vi "CreateFolder.vi"(4 "error in (no error)":errorcluster caption="エラー入力(エラーなし)", 7 "パス":path) -> (0 "error out":errorcluster caption="エラー出力", 3 "パス出力":path)   [LabVIEW 2015]
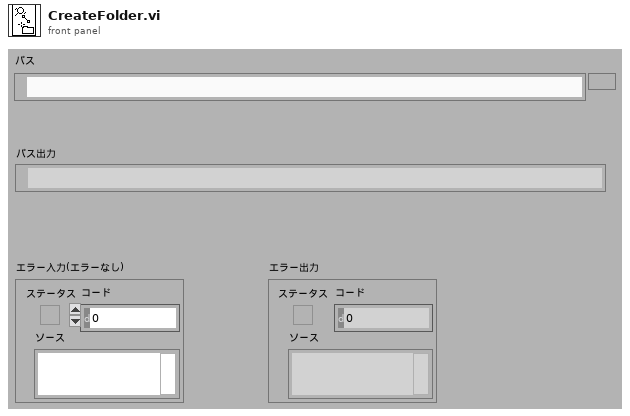
[diagram p1: front panel]
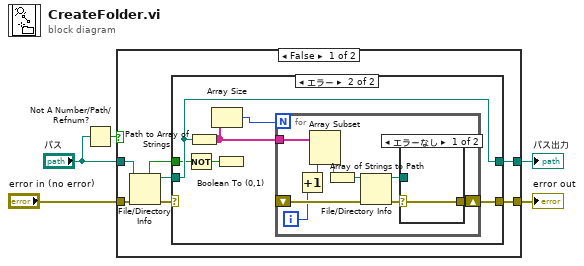
[diagram p0: block diagram]
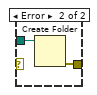
[diagram p3: hidden frame]
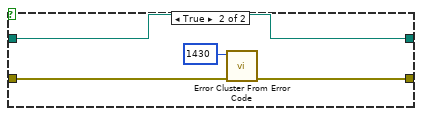
[diagram p4: hidden frame]
diagram:
  n1 = Not A Number/Path/Refnum?(number/path/refnum="パス") -> (NaN/Path/Refnum?=w5:bool)
  n2 = case shown="FALSE" w5 {
    tunnel: [w11 w36] -> w1
    tunnel: "error in (no error)" -> [w9 w34]
    tunnel: "パス" -> [w10 w33]
    tunnel: [w12 w33] -> w3
    frame False {
      n3 = File/Directory Info(path=w10, error in=w9) -> (path out=w7:path, directory=w6:bool, error out=w8:errorcluster)  [unwired: 4 out]
      n4 = case shown="エラー" w8 {
        selector: w8 -> [w13 _]
        tunnel: w7 -> [w14 w18]
        tunnel: [w14 w18] -> w12
        tunnel: [w13 w19] -> w11
        tunnel: w6 -> [_ w17]
        frame No Error {
        }
        frame Error {
          n5 = Not(x=w17) -> (.not. x?=w16:bool)
          n6 = Path to Array of Strings(0:w18) -> (2:w20:string[])  [unwired: 1 out]
          n7 = Array Size(array=w20) -> (size(s)=w15:i32)
          n8 = Boolean To (0,1)(Boolean=w16) -> ()  [unwired: 1 out]
          n9 = for {
            N: w15 -> [_]
            tunnel: w20 -> [w29]
            shift-right: [w23] -> w19
            shift-left: _ -> [w25]
            i -> [w21]
            n10 = Increment(x=w21) -> (x+1=w28:i32)
            n11 = Array Subset(array=w29, length=w28) -> (w27:string[])  [unwired: 1 in]
            n12 = Array of Strings to Path(0:w27) -> (2:w26:path)  [unwired: 1 in]
            n13 = File/Directory Info(path=w26, error in=w25) -> (path out=w22:path, error out=w24:errorcluster)  [unwired: 5 out]
            n14 = case shown="エラーなし" w24 {
              selector: w24 -> [w30 _]
              tunnel: [w30 w31] -> w23
              tunnel: w22 -> [_ w32]
              frame No Error {
              }
              frame Error {
                n15 = Create Folder(path (use dialog)=w32) -> (error out=w31:errorcluster)  [unwired: 1 in, 3 out]
              }
            }
          }
        }
      }
    }
    frame True {
      n16 = call <vilib>:"Error Cluster From Error Code.vi"("error in (no error)"=w34, "error code (0)"=1430) -> ("error out"=w36:errorcluster)  [unwired: 1 in, 6 out]
    }
  }
  "パス出力" <- w3
  "error out" <- w1
